vi "Translate Object.vi"(8 "error in (no error)":errorcluster, 10 "Translation":cluster{"X":sgl, "Y":sgl, "Z":sgl}, 11 "Scene.Object In":refnum<vi>) -> (0 "error out":errorcluster, 3 "Scene.Object Out":refnum<vi>)   [LabVIEW 2020, in "NI_3D Picture Control.lvlib"]
doc: "Translates an object in a 3D scene by the vector you specify. This VI performs a relative translation from the object's current position."
uses:
  <vilib>/picture/3D Picture Control/NI_3D Picture Control.lvlib
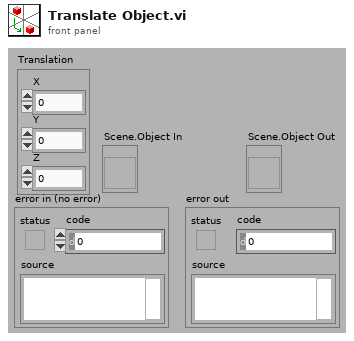
[diagram p1: front panel]
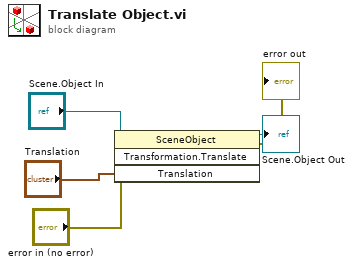
[diagram p0: block diagram]
diagram:
  n1 = invoke class="SceneObject" method="Transformation.Translate"(reference="Scene.Object In", error in="error in (no error)", "Translation"="Translation") -> (reference out=→"Scene.Object Out":refnum<vi>, error out=→"error out":errorcluster)  [unwired: 1 in, 2 out]
